vi "pitcherVictor.vi"   [LabVIEW 2011]
types:
  T1 = typedef "WPI_MotorControlDeviceRef.ctl" = cluster{"DeviceStatus":errorcluster, "Type":enum16{"PWM", "CAN"}, "PWM":cluster{"Digital Module":T2, "PWM Channel":T3, "DeadBand":T4}, "CAN":cluster{"Device Number":u8, "Control Mode":T5, "Semaphore":T6, "Max Vout":dbl}, "Invert":bool, "TransformRef":T7, "InvTransformRef":T7}
  T2 = typedef "FPGA_TypedefDigitalModule.ctl" = enum16{"Digital Module 1", "Digital Module 2"}
  T3 = typedef "FPGA_DIOPWMChannel.ctl" = enum8{"PWM 1", "PWM 2", "PWM 3", "PWM 4", "PWM 5", "PWM 6", "PWM 7", "PWM 8", "PWM 9", "PWM 10", "Invalid"}
  T4 = typedef "WPI_PWMDeadband.ctl" = cluster{"Name":string, "maxPositivePwm":i32, "minPositivePwm":i32, "centerPwm":i32, "maxNegativePwm":i32, "minNegativePwm":i32, "angularRange":u16}
  T5 = typedef "WPI_CANJaguar_ControlMode.ctl" = enum8{"Percent VBus", "Current", "Speed", "Position", "Voltage"}
  T6 = typedef "Semaphore RefNum" = refnum<k1>
  T7 = typedef "WPI_PWMTransform_ConPane.ctl" = refnum<vi>
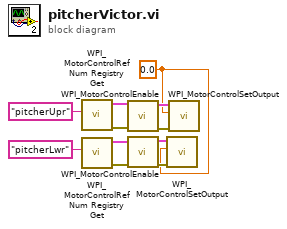
[diagram p0: block diagram]
diagram:
  w1 = 0.0 ("Output")
  n1 = call <vilib>:"WPI_MotorControlRefNum Registry Get.vi"("refnum name"="pitcherUpr") -> ("error out"=w9:errorcluster, "MotorControlDevRef"=w8:T1)  [unwired: 9 in]
  n2 = call <vilib>:"WPI_MotorControlRefNum Registry Get.vi"("refnum name"="pitcherLwr") -> ("error out"=w6:errorcluster, "MotorControlDevRef"=w7:T1)  [unwired: 9 in]
  n3 = call <vilib>:"WPI_MotorControlEnable.vi"("error in (no error)"=w9, "CAN Jaguar Ref"=w8) -> ("error out"=w5:errorcluster, "CAN Jaguar Ref Out"=w4:T1)  [unwired: 8 in]
  n4 = call <vilib>:"WPI_MotorControlEnable.vi"("error in (no error)"=w6, "CAN Jaguar Ref"=w7) -> ("error out"=w2:errorcluster, "CAN Jaguar Ref Out"=w3:T1)  [unwired: 8 in]
  n5 = call <vilib>:"WPI_MotorControlSetOutput.vi"("error in (no error)"=w2, "Output"=w1, "MotorControlDevRef"=w3) -> ()  [unwired: 7 in, 2 out]
  n6 = call <vilib>:"WPI_MotorControlSetOutput.vi"("error in (no error)"=w5, "Output"=w1, "MotorControlDevRef"=w4) -> ()  [unwired: 7 in, 2 out]
